vi "Initialize.vi"(8 "error in":errorcluster, 10 "parameters":variant, 11 "cDAQ in":refnum<class "PLTarget cDAQ.lvclass">) -> (0 "error out":errorcluster, 2 "summary":T2[](array[typedef]), 3 "data value reference":T1)   [LabVIEW 2013, in "PLTarget cDAQ.lvclass"]
doc: "This Vi initializes the data of a node its default state.\nThe object is not created inside of this ViI, beacuase it is created from a File depending on user selection."
uses:
  PLTarget cDAQ.lvclass
  <vilib>/NI/Configuration Framework/Node/Summary.ctl
  <vilib>/NI/Configuration Framework/Node/NodeRef.ctl
  <vilib>/NI/Configuration Framework/Node/NISE_CEF_Node.lvclass
  PLTarget cDAQ.lvclass/PLTarget cDAQ.ctl
  <vilib>/NI/Tag Bus Module Framework/root configuration/Target Types.ctl
  Framework Configuration Classes/target configuration/PL_Target Configuration.lvclass/PL_Target Configuration.ctl
  Configuration Editor/Classes/Targets/Targets.lvclass
  <vilib>/NI/Tag Bus Module Framework/root configuration/TBM configuration.lvclass
  Framework Configuration Classes/target configuration/PL_Target Configuration.lvclass
  <vilib>/NI/Configuration Framework/serializable configuration/NISE_CEF_serializable configuration.lvclass
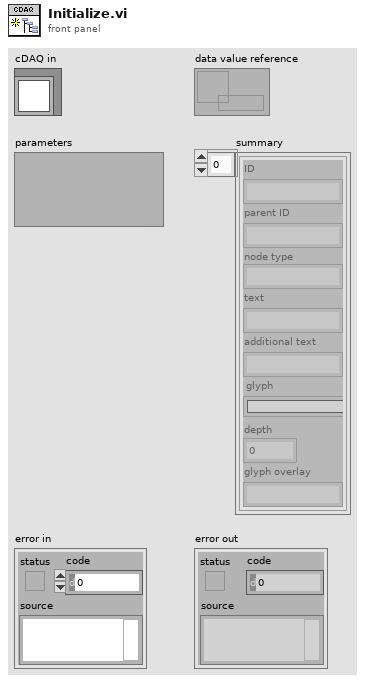
[diagram p1: front panel]
types:
  T1 = typedef "NISE_CEF_Node.lvclass/NodeRef.ctl" = refnum<data-value>
  T2 = typedef "NISE_CEF_Node.lvclass/Summary.ctl" = cluster{"ID":string, "parent ID":string, "node type":string, "text":string, "additional text":string, "glyph":string, "depth":i32, "glyph overlay":string}
  T3 = typedef "TBM configuration.lvclass/Target Types.ctl" = enum16{"Windows", "Mac", "Linux", "Linux RT ARM", "VxWorks", "Pharlap", "Other", "Linux RT x64"}
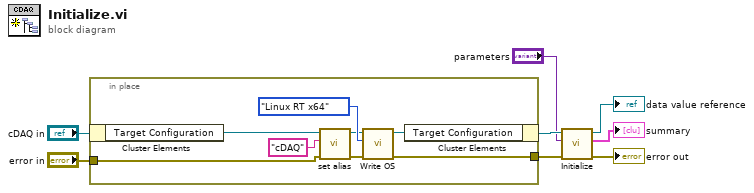
[diagram p0: block diagram]
diagram:
  n1 = in-place {
    in-place-border: [w14] -> w5
    in-place-border: "error in" -> [w15]
    n2 = in-place-cluster #1("cDAQ in") -> ("Target Configuration"=w9:refnum<class "PL_Target Configuration.lvclass">)
    n3 = call <vilib>:"set alias.vi"("error in"=w15, "alias"="cDAQ" ("name"), "configuration in"=w9) -> ("error out"=w11:errorcluster, "configuration out"=w12:refnum<class "PL_Target Configuration.lvclass">)  [unwired: 7 in]
    n4 = call "Write OS.vi"("error in"=w11, "Target Types"=Target_Types."Linux RT x64" ("OS"), "PL_Target Configuration in"=w12) -> ("error out"=w14:errorcluster, "PL_Target Configuration out"=w10:refnum<class "PL_Target Configuration.lvclass">)  [unwired: 7 in]
    n5 = in-place-cluster #1("Target Configuration"=w10) -> (w4:refnum<class "PLTarget cDAQ.lvclass">)
  }
  n6 = call-parent "Initialize.vi"("error in"=w5, "parameters"="parameters", "node in"=w4) -> ("error out"=→"error out":errorcluster, "summary"=→"summary":T2[], "data value reference"=→"data value reference":T1)  [unwired: 6 in]
